vi "Lakeshore_370_write.vi"   [LabVIEW 2016]
uses:
  Global/Global Variables/global.vi
  Instrument_Setup.vi
  Global/Global Variables/Data_Display_global.vi
panel:
  # "OFF"
  # "ON"
  # "OFF"
  # "ON"
  # "OFF"
  # "ON"
  # "OFF"
  # "ON"
  # "ON"
  # "OFF"
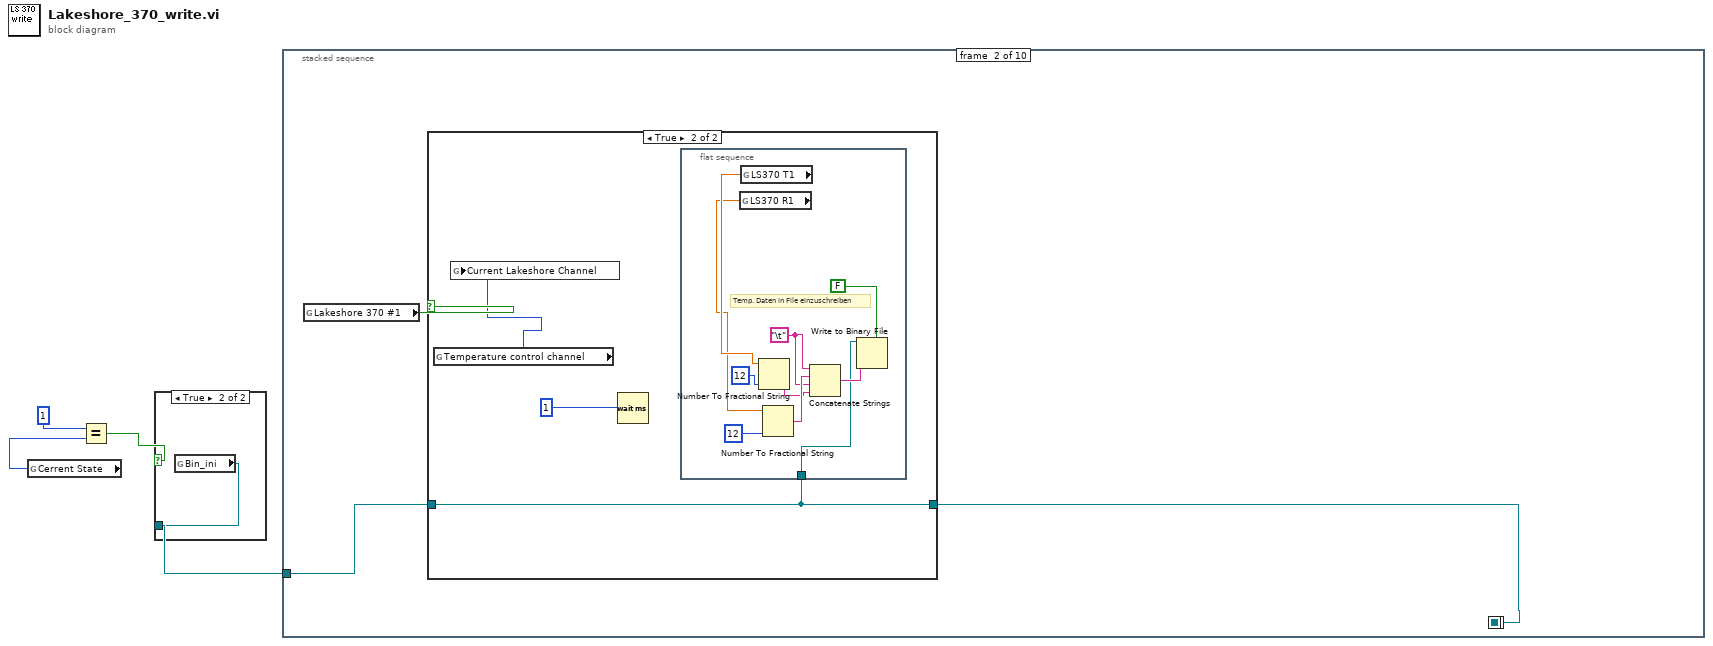
[diagram p0: block diagram]
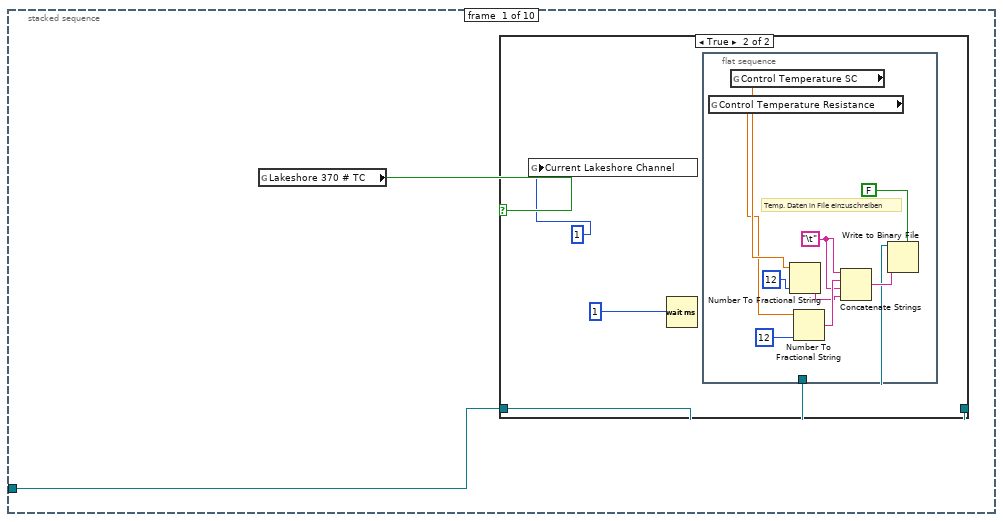
[diagram p2: hidden frame]
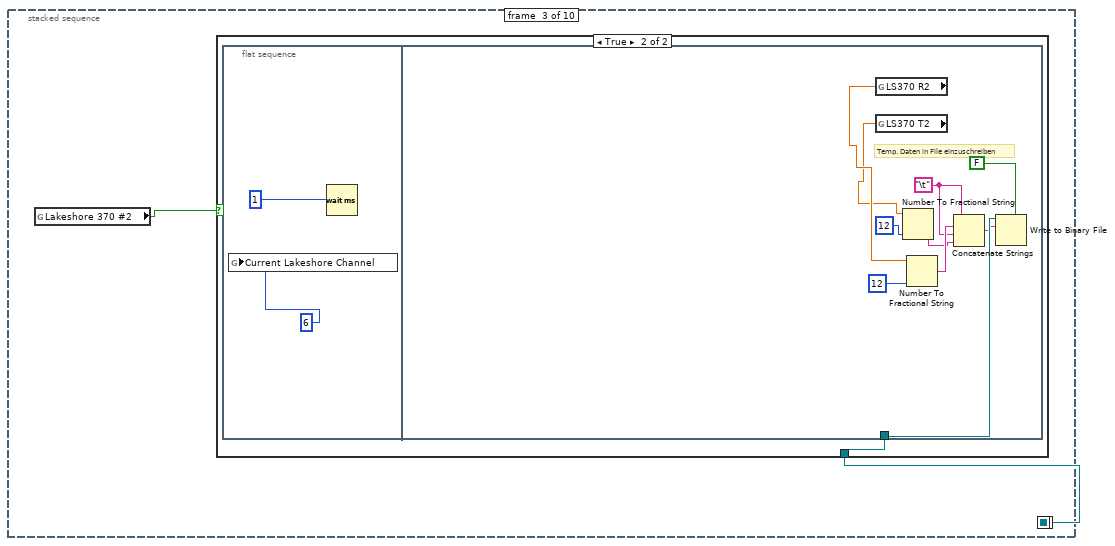
[diagram p5: hidden frame]
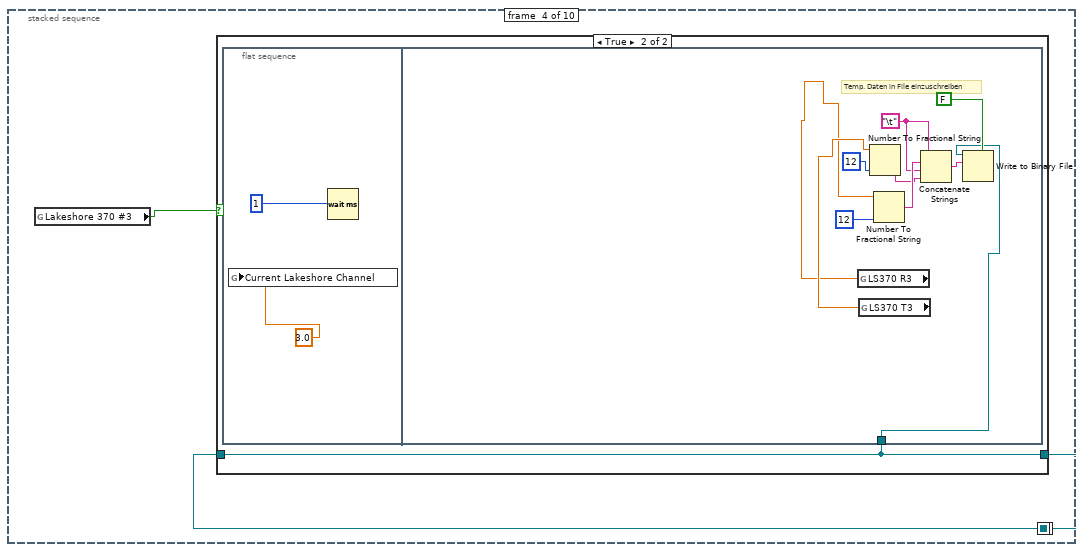
[diagram p7: hidden frame]
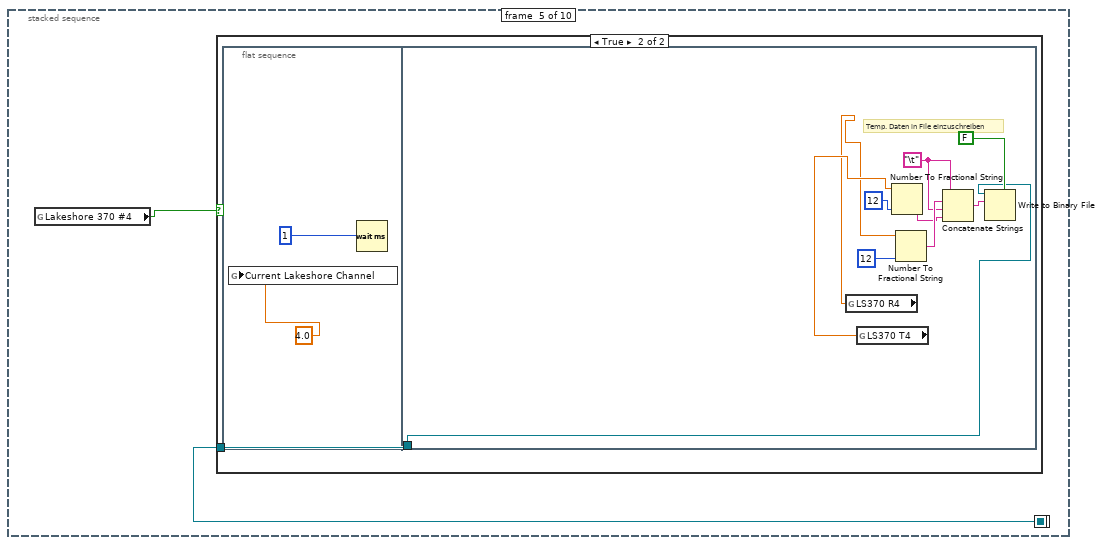
[diagram p9: hidden frame]
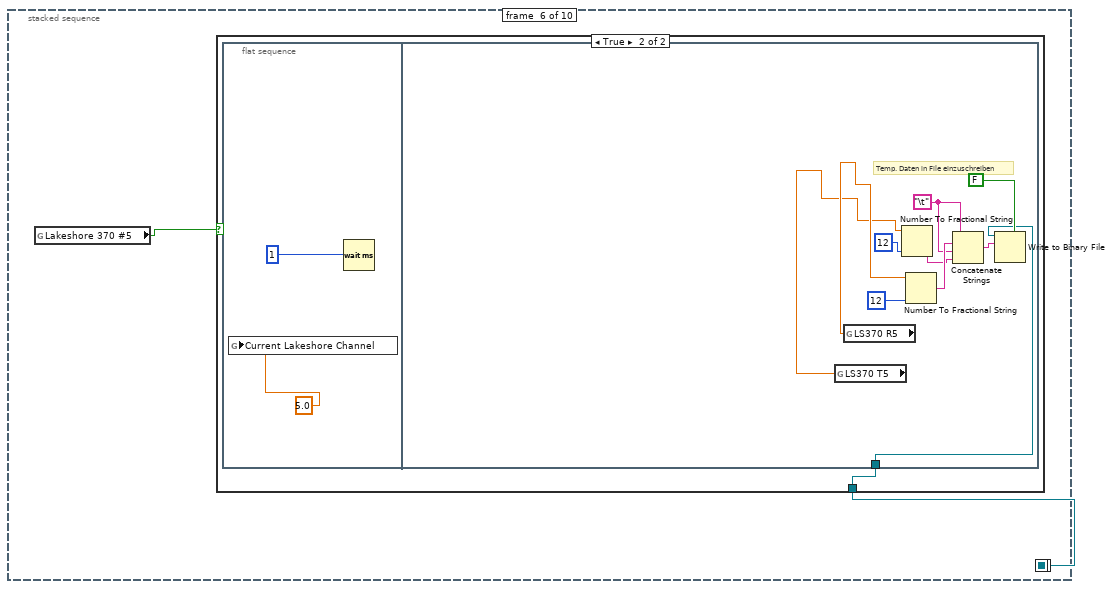
[diagram p11: hidden frame]
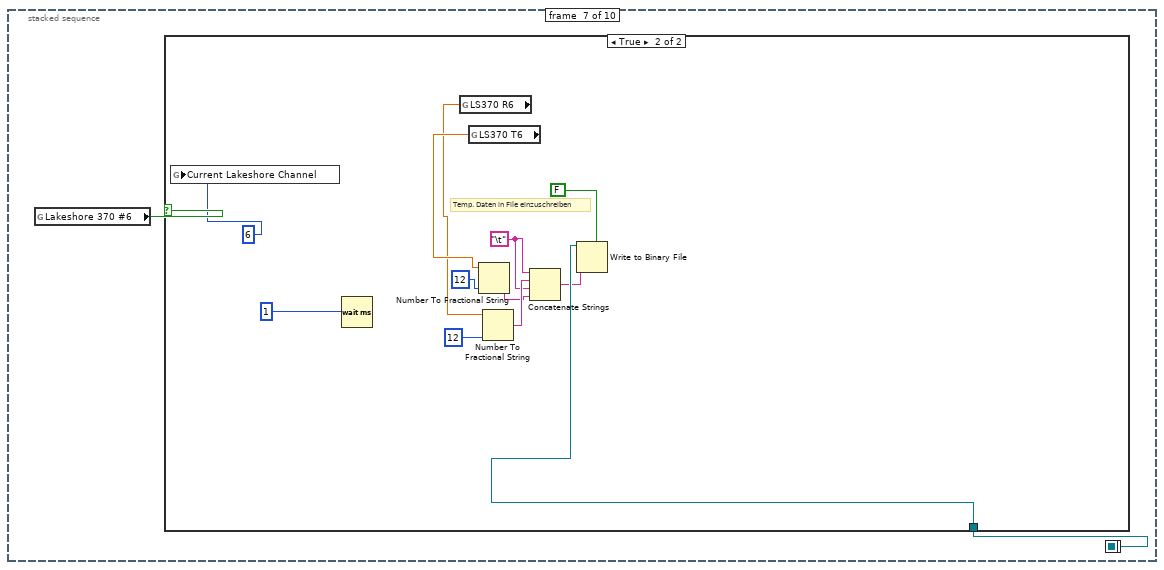
[diagram p13: hidden frame]
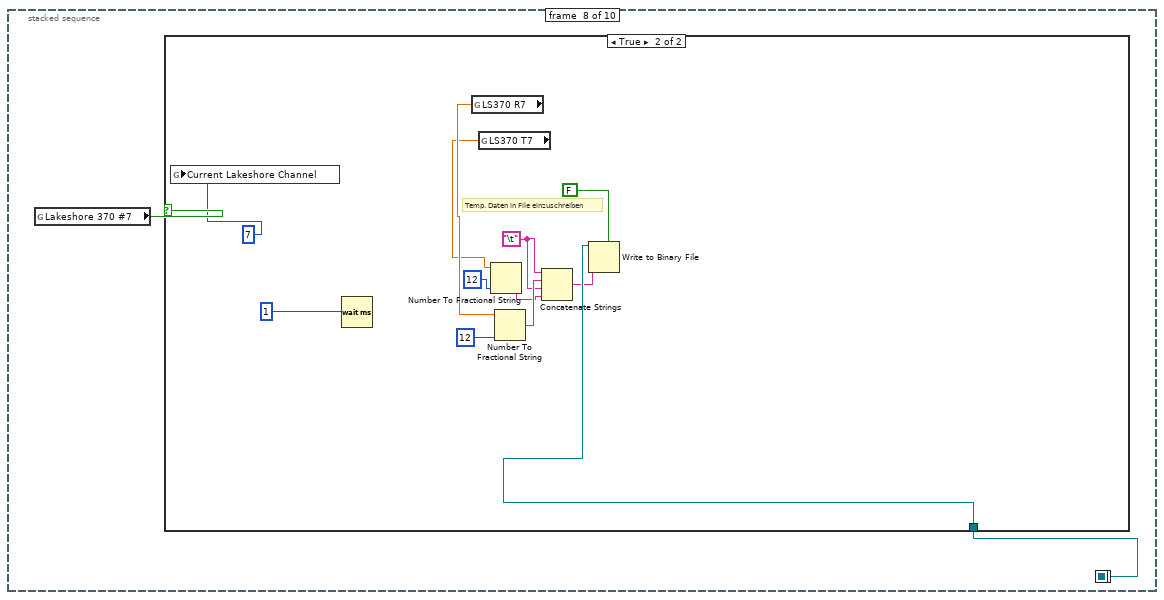
[diagram p15: hidden frame]
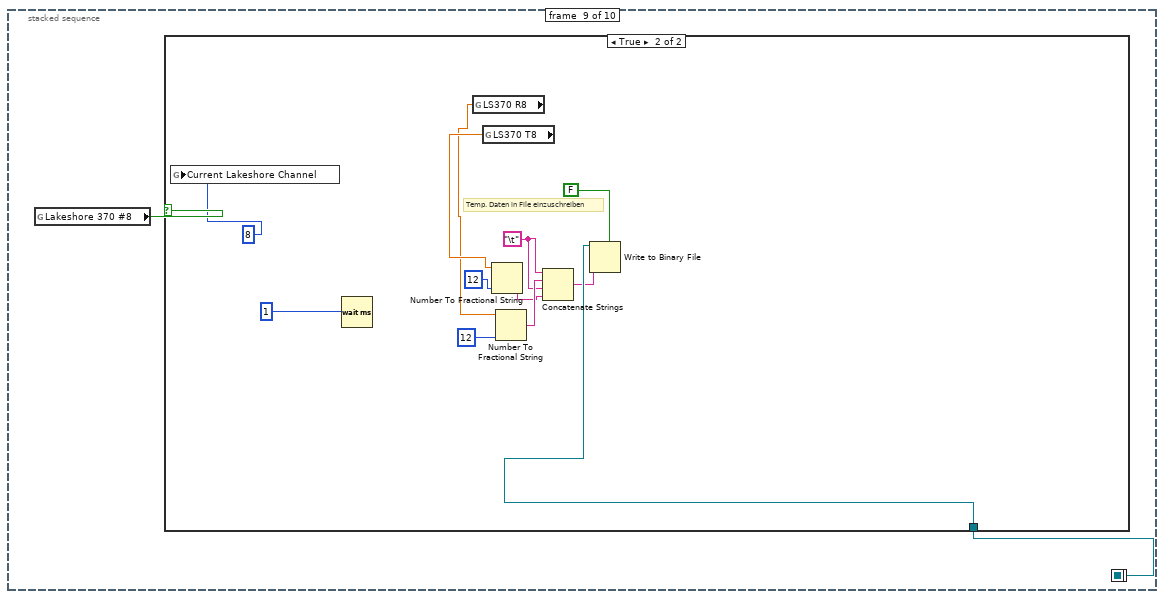
[diagram p17: hidden frame]
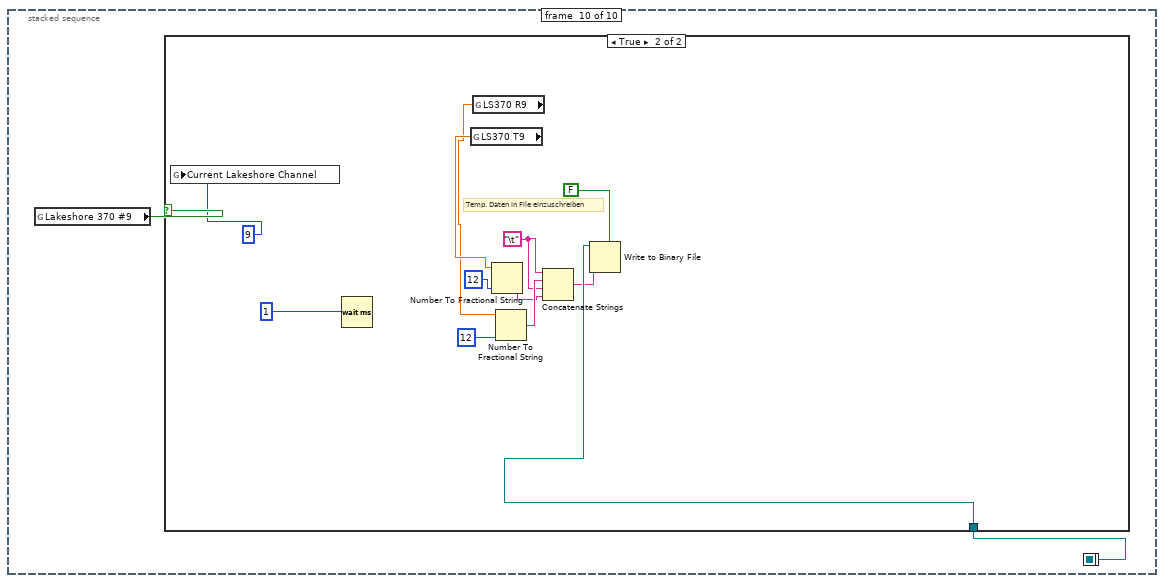
[diagram p19: hidden frame]
diagram:
  n1 = global read "global.vi" "Cerrent State"() -> (w3:i32)
  n2 = Equal?(x=1, y=w3) -> (x = y?=w2:bool)
  n3 = case shown="True" w2 {
    tunnel: [w5 w6] -> w1
    frame False {
      n4 = global read "Instrument_Setup.vi" "Bin_file"() -> (w5:refnum<file>)
    }
    frame True {
      n5 = global read "Instrument_Setup.vi" "Bin_ini"() -> (w6:refnum<file>)
    }
  }
  n6 = stacked-sequence {
    seq-local: [_ w24 _ _ _ _ _ _ _ _] -> [_ _ w40 w56 _ _ w102 w116 w130 w144]
    seq-local: [_ _ _ w55 _ _ _ _ _ _] -> [_ _ _ _ w72 _ _ _ _ _]
    seq-local: [_ _ _ _ w72 _ _ _ _ _] -> [_ _ _ _ _ w87 _ _ _ _]
    tunnel: w1 -> [w7 w23 _ _ _ _ _ _ _ _]
    frame #0 {
      n7 = global read "Instrument_Setup.vi" "Lakeshore 370 # TC"() -> (w8:bool)
      n8 = case shown="True" w8 {
        tunnel: w7 -> [w9 w12]
        tunnel: [w9 w12] -> _
        frame False {
        }
        frame True {
          n9 = global write "global.vi" "Current Lakeshore Channel"(1) -> ()
          n10 = Wait (ms)(milliseconds to wait=1) -> ()  [unwired: 1 out]
          n11 = flat-sequence {
            tunnel: w12 -> [w18]
            frame #0 {
              w16 = "\t"
              # "Temp. Daten in File einzuschreiben"
              n12 = global read "Data_Display_global.vi" "Control Temperature Resistance"() -> (w13:dbl)
              n13 = global read "Data_Display_global.vi" "Control Temperature SC"() -> (w14:dbl)
              n14 = Number To Fractional String(number=w14, precision (6)=i16 12) -> (F-format string=w15:string)  [unwired: 2 in]
              n15 = Number To Fractional String(number=w13, precision (6)=i16 12) -> (F-format string=w21:string)  [unwired: 2 in]
              n16 = Concatenate Strings(w16, w21, w16, w15) -> (w22:string)
              n17 = Write to Binary File ("Write File")(file (use dialog)=w18, data=w22, 5:FALSE ("prepend array or string size? (T)")) -> ()  [unwired: 3 in, 3 out]
            }
          }
        }
      }
    }
    frame #1 {
      n18 = global read "Instrument_Setup.vi" "Lakeshore 370 #1"() -> (w25:bool)
      n19 = case shown="True" w25 {
        tunnel: w23 -> [w26 w28]
        tunnel: [w26 w28] -> w24
        frame False {
        }
        frame True {
          n20 = global read "Instrument_Setup.vi" "Temperature control channel"() -> (w27:i32)
          n21 = global write "global.vi" "Current Lakeshore Channel"(w27) -> ()
          n22 = Wait (ms)(milliseconds to wait=1) -> ()  [unwired: 1 out]
          n23 = flat-sequence {
            tunnel: w28 -> [w30]
            frame #0 {
              w34 = "\t"
              # "Temp. Daten in File einzuschreiben"
              n24 = global read "Data_Display_global.vi" "LS370 R1"() -> (w31:dbl)
              n25 = global read "Data_Display_global.vi" "LS370 T1"() -> (w32:dbl)
              n26 = Number To Fractional String(number=w32, precision (6)=i16 12) -> (F-format string=w33:string)  [unwired: 2 in]
              n27 = Number To Fractional String(number=w31, precision (6)=i16 12) -> (F-format string=w38:string)  [unwired: 2 in]
              n28 = Concatenate Strings(w34, w38, w34, w33) -> (w39:string)
              n29 = Write to Binary File ("Write File")(file (use dialog)=w30, data=w39, 5:FALSE ("prepend array or string size? (T)")) -> ()  [unwired: 3 in, 3 out]
            }
          }
        }
      }
    }
    frame #2 {
      n30 = global read "Instrument_Setup.vi" "Lakeshore 370 #2"() -> (w41:bool)
      n31 = case shown="True" w41 {
        tunnel: w40 -> [_ w42]
        frame False {
        }
        frame True {
          n32 = flat-sequence {
            tunnel: w42 -> [w53]
            frame #0 {
              n33 = global write "global.vi" "Current Lakeshore Channel"(6) -> ()
              n34 = Wait (ms)(milliseconds to wait=1) -> ()  [unwired: 1 out]
            }
            frame #1 {
              w49 = "\t"
              # "Temp. Daten in File einzuschreiben"
              n35 = global read "Data_Display_global.vi" "LS370 R2"() -> (w46:dbl)
              n36 = global read "Data_Display_global.vi" "LS370 T2"() -> (w45:dbl)
              n37 = Number To Fractional String(number=w45, precision (6)=i16 12) -> (F-format string=w48:string)  [unwired: 2 in]
              n38 = Number To Fractional String(number=w46, precision (6)=i16 12) -> (F-format string=w52:string)  [unwired: 2 in]
              n39 = Concatenate Strings(w49, w52, w49, w48) -> (w47:string)
              n40 = Write to Binary File ("Write File")(file (use dialog)=w53, data=w47, 5:FALSE ("prepend array or string size? (T)")) -> ()  [unwired: 3 in, 3 out]
            }
          }
        }
      }
    }
    frame #3 {
      n41 = global read "Instrument_Setup.vi" "Lakeshore 370 #3"() -> (w57:bool)
      n42 = case shown="True" w57 {
        tunnel: w56 -> [w58 w59]
        tunnel: [w58 w59] -> w55
        frame False {
        }
        frame True {
          n43 = flat-sequence {
            tunnel: w59 -> [w64]
            frame #0 {
              n44 = global write "global.vi" "Current Lakeshore Channel"(3.0) -> ()
              n45 = Wait (ms)(milliseconds to wait=1) -> ()  [unwired: 1 out]
            }
            frame #1 {
              w67 = "\t"
              # "Temp. Daten in File einzuschreiben"
              n46 = global read "Data_Display_global.vi" "LS370 R3"() -> (w62:dbl)
              n47 = global read "Data_Display_global.vi" "LS370 T3"() -> (w63:dbl)
              n48 = Number To Fractional String(number=w63, precision (6)=i16 12) -> (F-format string=w66:string)  [unwired: 2 in]
              n49 = Number To Fractional String(number=w62, precision (6)=i16 12) -> (F-format string=w70:string)  [unwired: 2 in]
              n50 = Concatenate Strings(w67, w70, w67, w66) -> (w65:string)
              n51 = Write to Binary File ("Write File")(file (use dialog)=w64, data=w65, 5:FALSE ("prepend array or string size? (T)")) -> ()  [unwired: 3 in, 3 out]
            }
          }
        }
      }
    }
    frame #4 {
      n52 = global read "Instrument_Setup.vi" "Lakeshore 370 #4"() -> (w73:bool)
      n53 = case shown="True" w73 {
        tunnel: w72 -> [_ w74]
        frame False {
        }
        frame True {
          n54 = flat-sequence {
            tunnel: w74 -> [w79]
            frame #0 {
              n55 = global write "global.vi" "Current Lakeshore Channel"(4.0) -> ()
              n56 = Wait (ms)(milliseconds to wait=1) -> ()  [unwired: 1 out]
            }
            frame #1 {
              w82 = "\t"
              # "Temp. Daten in File einzuschreiben"
              n57 = global read "Data_Display_global.vi" "LS370 R4"() -> (w77:dbl)
              n58 = global read "Data_Display_global.vi" "LS370 T4"() -> (w78:dbl)
              n59 = Number To Fractional String(number=w78, precision (6)=i16 12) -> (F-format string=w81:string)  [unwired: 2 in]
              n60 = Number To Fractional String(number=w77, precision (6)=i16 12) -> (F-format string=w85:string)  [unwired: 2 in]
              n61 = Concatenate Strings(w82, w85, w82, w81) -> (w80:string)
              n62 = Write to Binary File ("Write File")(file (use dialog)=w79, data=w80, 5:FALSE ("prepend array or string size? (T)")) -> ()  [unwired: 3 in, 3 out]
            }
          }
        }
      }
    }
    frame #5 {
      n63 = global read "Instrument_Setup.vi" "Lakeshore 370 #5"() -> (w88:bool)
      n64 = case shown="True" w88 {
        tunnel: w87 -> [_ w89]
        frame False {
        }
        frame True {
          n65 = flat-sequence {
            tunnel: w89 -> [w94]
            frame #0 {
              n66 = global write "global.vi" "Current Lakeshore Channel"(5.0) -> ()
              n67 = Wait (ms)(milliseconds to wait=1) -> ()  [unwired: 1 out]
            }
            frame #1 {
              w97 = "\t"
              # "Temp. Daten in File einzuschreiben"
              n68 = global read "Data_Display_global.vi" "LS370 T5"() -> (w92:dbl)
              n69 = global read "Data_Display_global.vi" "LS370 R5"() -> (w93:dbl)
              n70 = Number To Fractional String(number=w92, precision (6)=i16 12) -> (F-format string=w96:string)  [unwired: 2 in]
              n71 = Number To Fractional String(number=w93, precision (6)=i16 12) -> (F-format string=w100:string)  [unwired: 2 in]
              n72 = Concatenate Strings(w97, w100, w97, w96) -> (w95:string)
              n73 = Write to Binary File ("Write File")(file (use dialog)=w94, data=w95, 5:FALSE ("prepend array or string size? (T)")) -> ()  [unwired: 3 in, 3 out]
            }
          }
        }
      }
    }
    frame #6 {
      n74 = global read "Instrument_Setup.vi" "Lakeshore 370 #6"() -> (w103:bool)
      n75 = case shown="True" w103 {
        tunnel: w102 -> [_ w113]
        frame False {
        }
        frame True {
          w107 = "\t"
          # "Temp. Daten in File einzuschreiben"
          n76 = global write "global.vi" "Current Lakeshore Channel"(6) -> ()
          n77 = Wait (ms)(milliseconds to wait=1) -> ()  [unwired: 1 out]
          n78 = global read "Data_Display_global.vi" "LS370 R6"() -> (w104:dbl)
          n79 = global read "Data_Display_global.vi" "LS370 T6"() -> (w105:dbl)
          n80 = Number To Fractional String(number=w105, precision (6)=i16 12) -> (F-format string=w106:string)  [unwired: 2 in]
          n81 = Number To Fractional String(number=w104, precision (6)=i16 12) -> (F-format string=w111:string)  [unwired: 2 in]
          n82 = Concatenate Strings(w107, w111, w107, w106) -> (w112:string)
          n83 = Write to Binary File ("Write File")(file (use dialog)=w113, data=w112, 5:FALSE ("prepend array or string size? (T)")) -> ()  [unwired: 3 in, 3 out]
        }
      }
    }
    frame #7 {
      n84 = global read "Instrument_Setup.vi" "Lakeshore 370 #7"() -> (w117:bool)
      n85 = case shown="True" w117 {
        tunnel: w116 -> [_ w127]
        frame False {
        }
        frame True {
          w121 = "\t"
          # "Temp. Daten in File einzuschreiben"
          n86 = global write "global.vi" "Current Lakeshore Channel"(7) -> ()
          n87 = Wait (ms)(milliseconds to wait=1) -> ()  [unwired: 1 out]
          n88 = global read "Data_Display_global.vi" "LS370 R7"() -> (w119:dbl)
          n89 = global read "Data_Display_global.vi" "LS370 T7"() -> (w118:dbl)
          n90 = Number To Fractional String(number=w118, precision (6)=i16 12) -> (F-format string=w120:string)  [unwired: 2 in]
          n91 = Number To Fractional String(number=w119, precision (6)=i16 12) -> (F-format string=w125:string)  [unwired: 2 in]
          n92 = Concatenate Strings(w121, w125, w121, w120) -> (w126:string)
          n93 = Write to Binary File ("Write File")(file (use dialog)=w127, data=w126, 5:FALSE ("prepend array or string size? (T)")) -> ()  [unwired: 3 in, 3 out]
        }
      }
    }
    frame #8 {
      n94 = global read "Instrument_Setup.vi" "Lakeshore 370 #8"() -> (w131:bool)
      n95 = case shown="True" w131 {
        tunnel: w130 -> [_ w141]
        frame False {
        }
        frame True {
          w135 = "\t"
          # "Temp. Daten in File einzuschreiben"
          n96 = global write "global.vi" "Current Lakeshore Channel"(8) -> ()
          n97 = Wait (ms)(milliseconds to wait=1) -> ()  [unwired: 1 out]
          n98 = global read "Data_Display_global.vi" "LS370 R8"() -> (w132:dbl)
          n99 = global read "Data_Display_global.vi" "LS370 T8"() -> (w133:dbl)
          n100 = Number To Fractional String(number=w133, precision (6)=i16 12) -> (F-format string=w134:string)  [unwired: 2 in]
          n101 = Number To Fractional String(number=w132, precision (6)=i16 12) -> (F-format string=w139:string)  [unwired: 2 in]
          n102 = Concatenate Strings(w135, w139, w135, w134) -> (w140:string)
          n103 = Write to Binary File ("Write File")(file (use dialog)=w141, data=w140, 5:FALSE ("prepend array or string size? (T)")) -> ()  [unwired: 3 in, 3 out]
        }
      }
    }
    frame #9 {
      n104 = global read "Instrument_Setup.vi" "Lakeshore 370 #9"() -> (w145:bool)
      n105 = case shown="True" w145 {
        tunnel: w144 -> [_ w155]
        frame False {
        }
        frame True {
          w149 = "\t"
          # "Temp. Daten in File einzuschreiben"
          n106 = global write "global.vi" "Current Lakeshore Channel"(9) -> ()
          n107 = Wait (ms)(milliseconds to wait=1) -> ()  [unwired: 1 out]
          n108 = global read "Data_Display_global.vi" "LS370 T9"() -> (w147:dbl)
          n109 = global read "Data_Display_global.vi" "LS370 R9"() -> (w146:dbl)
          n110 = Number To Fractional String(number=w147, precision (6)=i16 12) -> (F-format string=w148:string)  [unwired: 2 in]
          n111 = Number To Fractional String(number=w146, precision (6)=i16 12) -> (F-format string=w153:string)  [unwired: 2 in]
          n112 = Concatenate Strings(w149, w153, w149, w148) -> (w154:string)
          n113 = Write to Binary File ("Write File")(file (use dialog)=w155, data=w154, 5:FALSE ("prepend array or string size? (T)")) -> ()  [unwired: 3 in, 3 out]
        }
      }
    }
  }
